vi "DHE_exec_system.vi"(7 "wait until completion? (T)":bool=TRUE, 8 "error in (no error)":errorcluster, 9 "command line":string, 10 "working directory":path=path "") -> (0 "error out":errorcluster, 2 "response":string)   [LabVIEW 2016]
uses:
  <vilib>/Utility/error.llb/DialogType.ctl
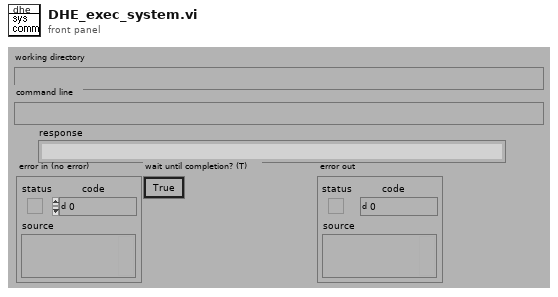
[diagram p1: front panel]
types:
  T1 = typedef "DialogType.ctl" = u16
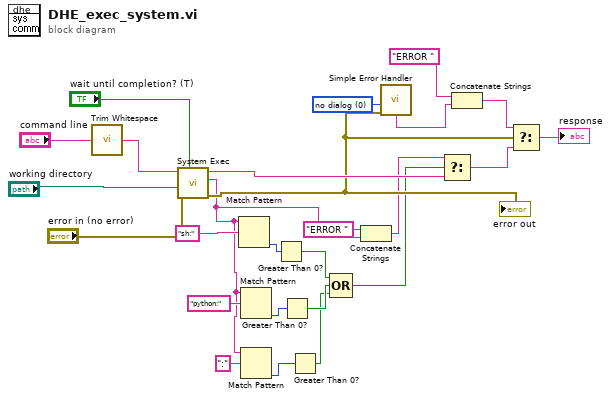
[diagram p0: block diagram]
diagram:
  w23 = T1 0 items=["no dialog", "OK message", "continue or stop message", "OK message + warnings", "continue/stop + warnings"] ("type of dialog (OK msg:1)")
  n1 = call <vilib>:"Trim Whitespace.vi"("string"="command line") -> ("trimmed string"=w7:string)  [unwired: 1 in]
  n2 = call <vilib>:"System Exec.vi"("wait until completion? (T)"="wait until completion? (T)", "error in (no error)"="error in (no error)", "working directory"="working directory", "command line"=w7) -> ("error out"=w22:errorcluster, "standard error"=w3:string, "standard output"=w26:string)  [unwired: 2 in, 3 out]
  "error out" <- w22
  n3 = Match Pattern(string=w3, regular expression="sh:") -> (offset past match=w19:i32)  [unwired: 4 out]
  n4 = Match Pattern(string=w3, regular expression="python:") -> (offset past match=w17:i32)  [unwired: 4 out]
  n5 = Match Pattern(string=w3, regular expression=":") -> (offset past match=w2:i32)  [unwired: 4 out]
  n6 = Greater Than 0?(x=w19) -> (x > 0?=w16:bool)
  n7 = Greater Than 0?(x=w17) -> (x > 0?=w15:bool)
  n8 = Greater Than 0?(x=w2) -> (x > 0?=w1:bool)
  n9 = Compound Arithmetic op=OR(w16, w15, w1) -> (w14:bool)
  n10 = Concatenate Strings("ERROR " ("string"), w3) -> (w9:string)
  n11 = call <vilib>:"Simple Error Handler.vi"("type of dialog (OK msg:1)"=w23, "error in (no error)"=w22) -> ("message"=w11:string)  [unwired: 7 out]
  n12 = Select(t=w9, s=w14, f=w26) -> (s? t:f=w13:string)
  n13 = Concatenate Strings("ERROR " ("string"), w11) -> (w10:string)
  n14 = Select(t=w10, s=w22, f=w13) -> (s? t:f=→"response":string)
